vi "main_create_environment.vi"(5 "Ready?":refnum<vi>, 6 "Storage?":refnum<vi>, 7 "Methane?":refnum<vi>, 8 "Running?":refnum<vi>, 9 "Directory":refnum<vi>, 10 "Create":refnum<vi>, 11 "Environtment Tree":refnum<vi>) -> ()   [LabVIEW 2019]
uses:
  lib/libSimulationControl/libSimulationControl.lvlib
panel:
  # "*******************************************************************\nBiogas Plant Control\n\nAuthor: Paul Zügel\nGCSC-Frankfurt am Main 2020\n\n*******************************************************************"
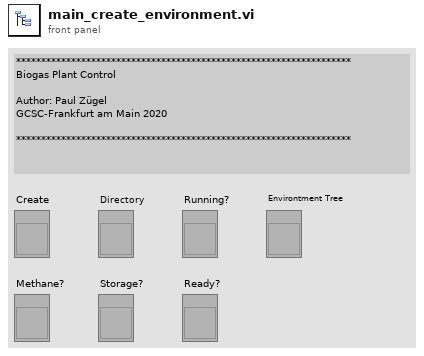
[diagram p1: front panel]
types:
  T1 = cluster{"filename without extension":string, "Child Text":string[], "Child Tag":string, i32, "Child Only?":bool, "Glyph Index":i32}[]
  T2 = enum8{"Enabled", "Disabled", "Disabled and Grayed Out"}
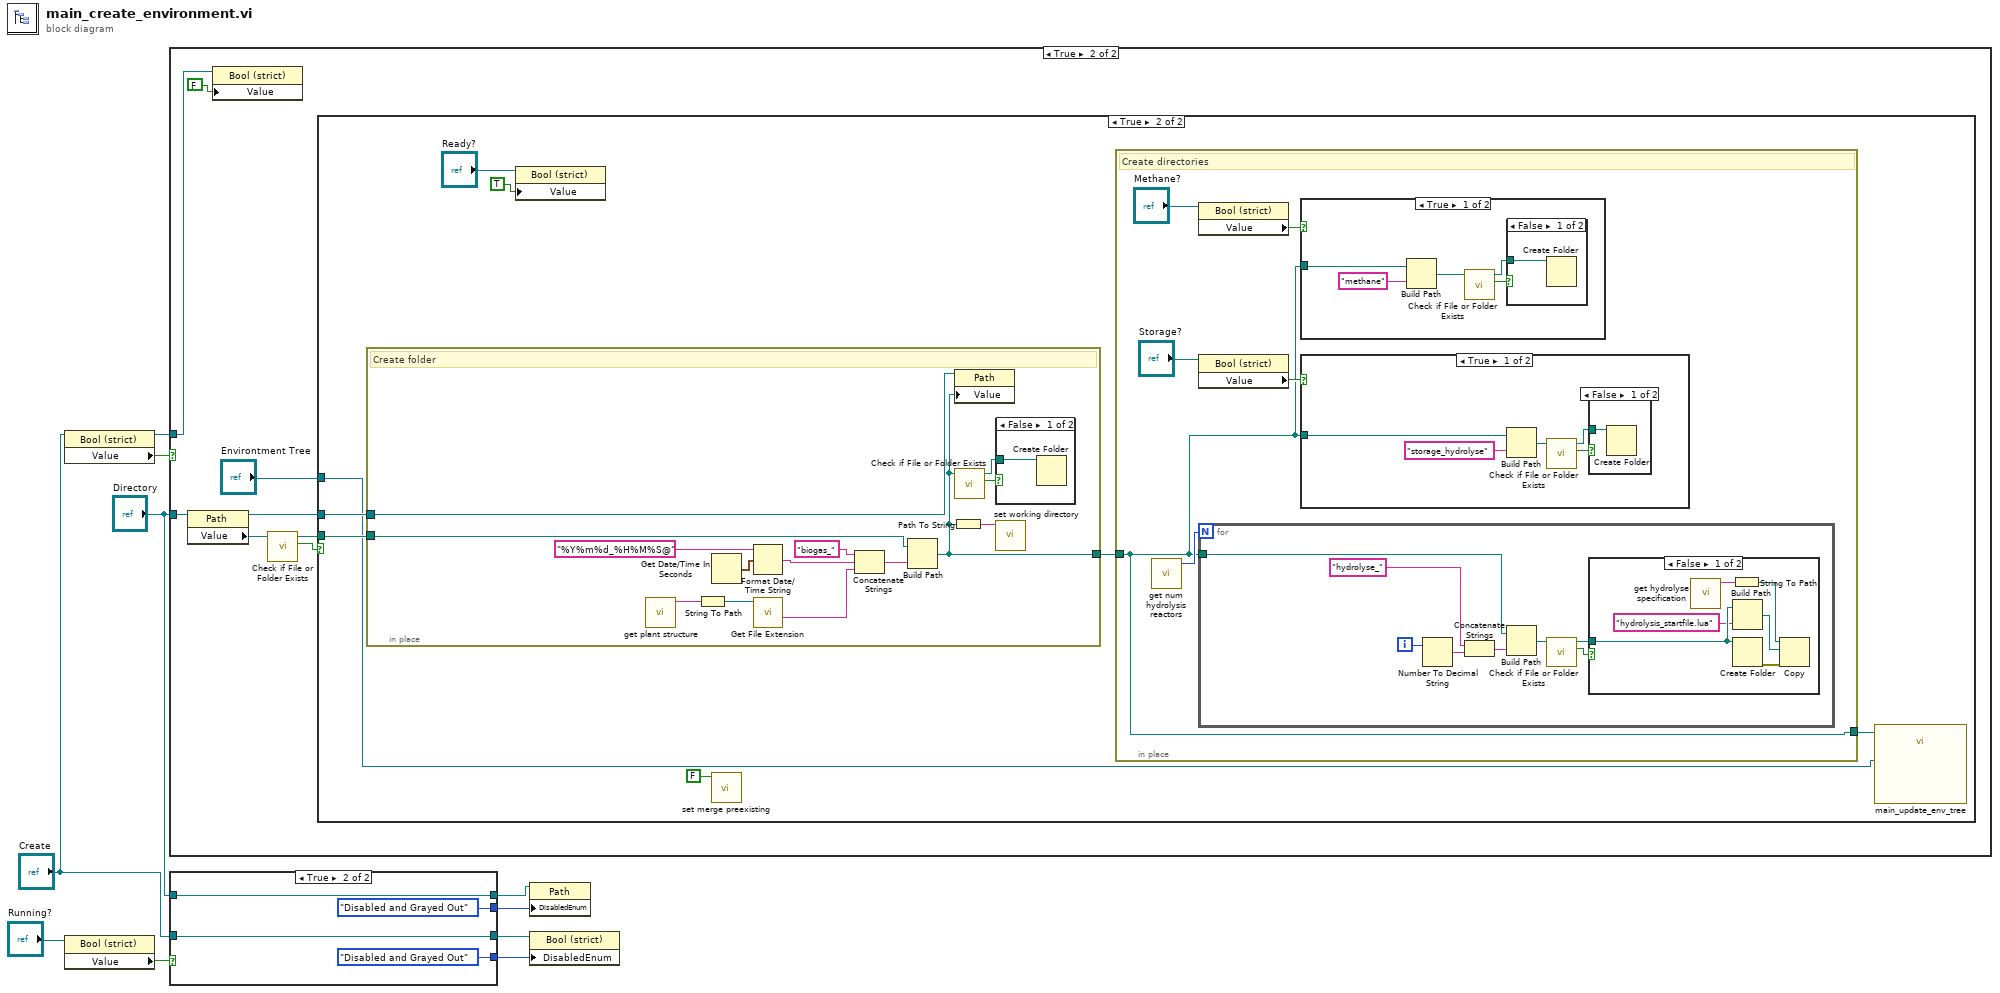
[diagram p0: block diagram]
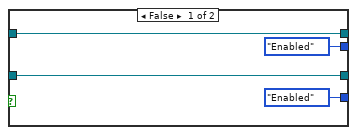
[diagram p2: hidden frame]
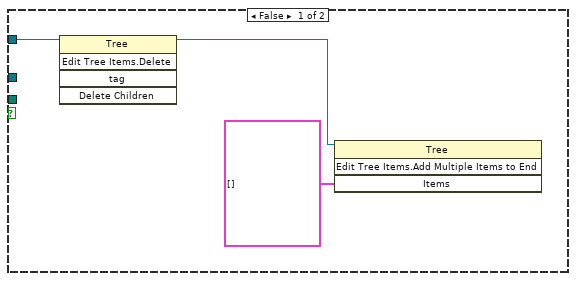
[diagram p4: hidden frame]
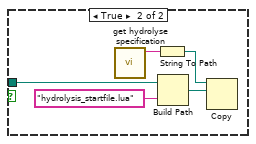
[diagram p6: hidden frame]
diagram:
  n1 = property class="Bool (strict)"(reference="Create") -> (reference out=w9:refnum<vi>, "Value"=w10:bool)  [unwired: 1 in, 1 out]
  n2 = property on="Property Node" class="Bool (strict)"(reference="Running?") -> ("Value"=w7:bool)  [unwired: 1 in, 2 out]
  n3 = case shown="True" w10 {
    tunnel: w9 -> [_ w15]
    tunnel: "Directory" -> [_ w13]
    frame False {
    }
    frame True {
      n4 = property class="Path"(reference=w13) -> (reference out=w12:refnum<vi>, "Value"=w16:path)  [unwired: 1 in, 1 out]
      n5 = property class="Bool (strict)"(reference=w15, "Value"=FALSE) -> ()  [unwired: 1 in, 2 out]
      n6 = call <vilib>:"Check if File or Folder Exists.vi"("path"=w16) -> ("file or folder exists?"=w18:bool, "dup path"=w17:path)  [unwired: 8 in, 1 out]
      n7 = case shown="True" w18 {
        tunnel: w17 -> [_ w29]
        tunnel: w12 -> [_ w25]
        tunnel: "Environtment Tree" -> [w19 w22]
        frame False {
          n8 = invoke class="Tree" method="Edit Tree Items.Delete"(reference=w19) -> (reference out=w20:refnum<vi>)  [unwired: 4 in, 4 out]
          n9 = invoke on="Invoke Node" class="Tree" method="Edit Tree Items.Add Multiple Items to End"(reference=w20, "Items"=T1 []) -> ()  [unwired: 2 in, 4 out]
        }
        frame True {
          n10 = in-place {
            in-place-border: w29 -> [w40]
            in-place-border: [w35] -> w28
            in-place-border: w25 -> [w36]
            # "Create folder"
            n11 = call "get plant structure.vi"() -> ("function return"=w38:string)  [unwired: 10 in, 1 out]
            n12 = String To Path(string=w38) -> (path=w37:path)
            n13 = Get Date/Time In Seconds() -> (seconds since 1Jan1904=w34:timestamp)
            n14 = Format Date/Time String(time format string (%c)="%Y%m%d_%H%M%S@", seconds (now)=w34) -> (date/time string=w31:string)  [unwired: 1 in]
            n15 = call <vilib>:"Get File Extension.vi"("file"=w37) -> ("filename without extension"=w30:string)  [unwired: 6 in, 4 out]
            n16 = Concatenate Strings("biogas_" ("string"), w31, w30) -> (w39:string)
            n17 = Build Path(base path=w40, name or relative path=w39) -> (appended path=w35:path)
            n18 = Path To String(path=w35) -> (string=w41:string)
            n19 = property class="Path"(reference=w36, "Value"=w35) -> ()  [unwired: 1 in, 2 out]
            n20 = call <vilib>:"Check if File or Folder Exists.vi"("path"=w35) -> ("file or folder exists?"=w43:bool, "dup path"=w42:path)  [unwired: 8 in, 1 out]
            n21 = case shown="False" w43 {
              tunnel: w42 -> [w44 _]
              frame False {
                n22 = Create Folder(path (use dialog)=w44) -> ()  [unwired: 2 in, 3 out]
              }
              frame True {
              }
            }
            n23 = call "set working directory.vi"("dir"=w41) -> ()  [unwired: 10 in, 1 out]
          }
          n24 = property class="Bool (strict)"(reference="Ready?", "Value"=TRUE) -> ()  [unwired: 1 in, 2 out]
          n25 = call "set merge preexisting.vi"("merge"=FALSE) -> ()  [unwired: 10 in, 1 out]
          n26 = in-place {
            in-place-border: w28 -> [w45]
            in-place-border: [w45] -> w23
            # "Create directories"
            n27 = call "get num hydrolysis reactors.vi"() -> ("function return"=w46:i32)  [unwired: 10 in, 1 out]
            n28 = property class="Bool (strict)"(reference="Methane?") -> ("Value"=w47:bool)  [unwired: 1 in, 2 out]
            n29 = property class="Bool (strict)"(reference="Storage?") -> ("Value"=w48:bool)  [unwired: 1 in, 2 out]
            n30 = for {
              N: w46 -> [_]
              tunnel: w45 -> [w58]
              i -> [w57]
              n31 = Number To Decimal String(number=w57) -> (decimal integer string=w51:string)  [unwired: 1 in]
              n32 = Concatenate Strings("hydrolyse_" ("string"), w51) -> (w52:string)
              n33 = Build Path(base path=w58, name or relative path=w52) -> (appended path=w56:path)
              n34 = call <vilib>:"Check if File or Folder Exists.vi"("path"=w56) -> ("file or folder exists?"=w55:bool, "dup path"=w54:path)  [unwired: 8 in, 1 out]
              n35 = case shown="False" w55 {
                tunnel: w54 -> [w61 w65]
                frame False {
                  n36 = call "get hydrolyse specification.vi"() -> ("function return"=w64:string)  [unwired: 10 in, 1 out]
                  n37 = String To Path(string=w64) -> (path=w62:path)
                  n38 = Build Path(base path=w61, name or relative path="hydrolysis_startfile.lua") -> (appended path=w59:path)
                  n39 = Create Folder(path (use dialog)=w61) -> (error out=w63:errorcluster)  [unwired: 2 in, 2 out]
                  n40 = Copy(8:w63, 10:w59, 11:w62) -> ()  [unwired: 2 in, 3 out]
                }
                frame True {
                  n41 = call "get hydrolyse specification.vi"() -> ("function return"=w69:string)  [unwired: 10 in, 1 out]
                  n42 = String To Path(string=w69) -> (path=w68:path)
                  n43 = Build Path(base path=w65, name or relative path="hydrolysis_startfile.lua") -> (appended path=w66:path)
                  n44 = Copy(10:w66, 11:w68) -> ()  [unwired: 3 in, 3 out]
                }
              }
            }
            n45 = case shown="True" w47 {
              tunnel: w45 -> [w74 _]
              frame True {
                n46 = Build Path(base path=w74, name or relative path="methane") -> (appended path=w72:path)
                n47 = call <vilib>:"Check if File or Folder Exists.vi"("path"=w72) -> ("file or folder exists?"=w71:bool, "dup path"=w70:path)  [unwired: 8 in, 1 out]
                n48 = case shown="False" w71 {
                  tunnel: w70 -> [w75 _]
                  frame False {
                    n49 = Create Folder(path (use dialog)=w75) -> ()  [unwired: 2 in, 3 out]
                  }
                  frame True {
                  }
                }
              }
              frame False {
              }
            }
            n50 = case shown="True" w48 {
              tunnel: w45 -> [w80 _]
              frame True {
                n51 = Build Path(base path=w80, name or relative path="storage_hydrolyse") -> (appended path=w78:path)
                n52 = call <vilib>:"Check if File or Folder Exists.vi"("path"=w78) -> ("file or folder exists?"=w77:bool, "dup path"=w76:path)  [unwired: 8 in, 1 out]
                n53 = case shown="False" w77 {
                  tunnel: w76 -> [w81 _]
                  frame False {
                    n54 = Create Folder(path (use dialog)=w81) -> ()  [unwired: 2 in, 3 out]
                  }
                  frame True {
                  }
                }
              }
              frame False {
              }
            }
          }
          n55 = call "main_update_env_tree.vi"("Env. Tree"=w22, "Env_path"=w23) -> ()  [unwired: 10 in]
        }
      }
    }
  }
  n56 = case shown="True" w7 {
    tunnel: "Create" -> [w85 w89]
    tunnel: "Directory" -> [w84 w88]
    tunnel: [w85 w89] -> w4
    tunnel: [w84 w88] -> w3
    tunnel: [T2."Enabled" ("Disabled") T2."Disabled and Grayed Out" ("Disabled")] -> w2
    tunnel: [T2."Enabled" ("Disabled") T2."Disabled and Grayed Out" ("Disabled")] -> w1
    frame False {
    }
    frame True {
    }
  }
  n57 = property class="Path"(reference=w3, "DisabledEnum"=w2) -> ()  [unwired: 1 in, 2 out]
  n58 = property class="Bool (strict)"(reference=w4, "DisabledEnum"=w1) -> ()  [unwired: 1 in, 2 out]
